vi "NodesFG.vi"(10 "Node Name":string, 11 "Function":string) -> (1 "key not found?":bool, 2 "Value":dbl, 3 "Node List":string[](array[string]))   [LabVIEW 2021]
uses:
  <vilib>/numeric/Random Number (Range) DBL.vi
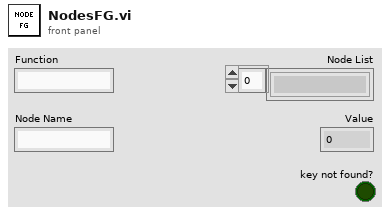
[diagram p1: front panel]
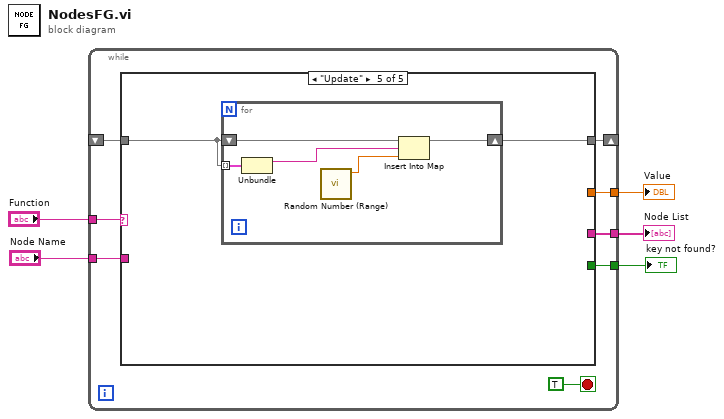
[diagram p0: block diagram]
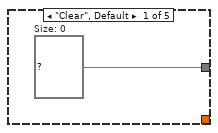
[diagram p2: hidden frame]
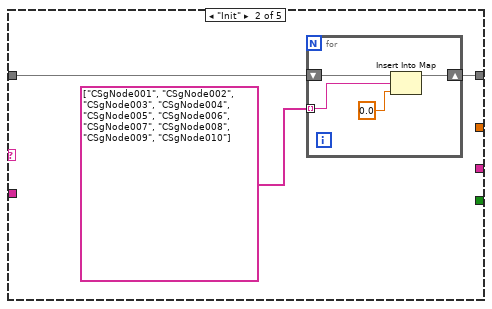
[diagram p3: hidden frame]
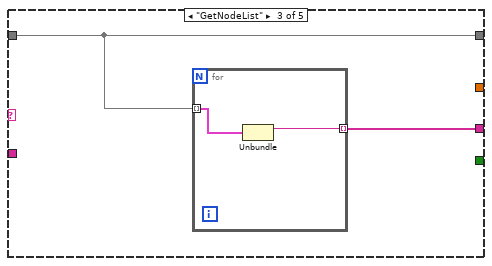
[diagram p4: hidden frame]
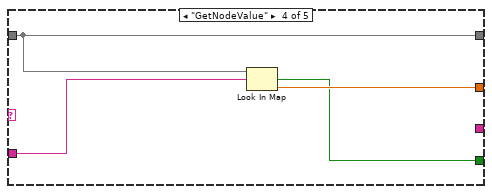
[diagram p5: hidden frame]
diagram:
  n1 = while {
    tunnel: "Function" -> [w12]
    shift-right: [w11] -> _
    shift-left: _ -> [w10]
    tunnel: [w9] -> w4
    tunnel: "Node Name" -> [w8]
    tunnel: [w7] -> w2
    tunnel: [w6] -> w1
    stop <- TRUE stop-if-true
    n2 = case shown="\"Update\"" w12 {
      tunnel: [w14 w16 w23 w29 w30] -> w11
      tunnel: w10 -> [_ w15 w23 w29 w31]
      tunnel: [_ _ w22 _ _] -> w9
      tunnel: w8 -> [_ _ _ w28 _]
      tunnel: [_ _ _ w27 _] -> w7
      tunnel: [_ _ _ w26 _] -> w6
      frame "Clear", Default {
        w14 = map{string, dbl} {}  # Size: 0
      }
      frame "Init" {
        n3 = for {
          shift-right: [w21] -> w16
          shift-left: w15 -> [w20]
          tunnel: string[] ["CSgNode001", "CSgNode002", "CSgNode003", "CSgNode004", "CSgNode005", "CSgNode006", "CSgNode007", "CSgNode008", "CSgNode009", "CSgNode010"] -> [w18] mode=indexing
          n4 = Insert Into Map(map in=w20, key=w18, value=0.0) -> (map out=w21:map{string, dbl})  [unwired: 2 out]
        }
      }
      frame "GetNodeList" {
        n5 = for {
          tunnel: w23 -> [w25] mode=indexing
          tunnel: [w24] -> w22 mode=indexing
          n6 = Unbundle(w25) -> (w24:string)  [unwired: 1 out]
        }
      }
      frame "GetNodeValue" {
        n7 = Look In Map(map=w29, key=w28) -> (key not found?=w26:bool, value=w27:dbl)  [unwired: 1 in]
      }
      frame "Update" {
        n8 = for {
          tunnel: w31 -> [w36] mode=indexing
          shift-right: [w34] -> w30
          shift-left: w31 -> [w35]
          n9 = Unbundle(w36) -> (w32:string)  [unwired: 1 out]
          n10 = call-poly <vilib>:"Random Number (Range).vi"() -> ("number"=w33:dbl)  [unwired: 11 in]
          n11 = Insert Into Map(map in=w35, key=w32, value=w33) -> (map out=w34:map{string, dbl})  [unwired: 2 out]
        }
      }
    }
  }
  "Node List" <- w4
  "Value" <- w2
  "key not found?" <- w1
